vi "grapher.vi"(0 "Eventnum refnum":refnum<vi>, 5 "Frequency refnum":refnum<vi>, 7 "Stop signaller":refnum<class "Signaller.lvclass">, 9 "Polarization refnum":refnum<vi>, 11 "Rate refnum":refnum<vi>) -> ()   [LabVIEW 2015]
uses:
  Motor controller/Signaller/Signaller.lvclass
panel:
  in  "Focus range":dbl=0.1 min=0.001 step=0.1 format="%.3g"
  in  "Focus on current":bool
  in  "Scale for negative":bool
  in  "Scale for positive":bool
  in  "Autoscale polarization":bool=TRUE
  in  "Min polarization":dbl step=0.1 format="%.3g"
  in  "Max polarization":dbl=1.0 step=0.1 format="%.3g"
  in  "Add 1 hour":bool
  in  "1 hour":bool
  in  "30 minutes":bool
  in  "10 minutes":bool
  in  "5 minutes":bool
  in  "1 minute":bool
  in  "Time scale (min)":i64=1 min=1 step=1
  in  "Data output file":path
  out "Data points":i32
  out "Polarization vs frequency":cluster{dbl, dbl}[](graph)
  out "Rate vs time":cluster{"Value":i64, "Value":dbl}[](graph)
  out "Frequency vs time":cluster{"Value":i64, "Value":dbl}[](graph)
  out "Polarization vs time":cluster{i64, dbl}[](graph)
  out "Rate":dbl
  out "Polarization":dbl
  out "Frequency":dbl
  out "Eventnum":i64
  # "Advanced controls"
  # "Graph polarization scale"
  # "Graph time scale"
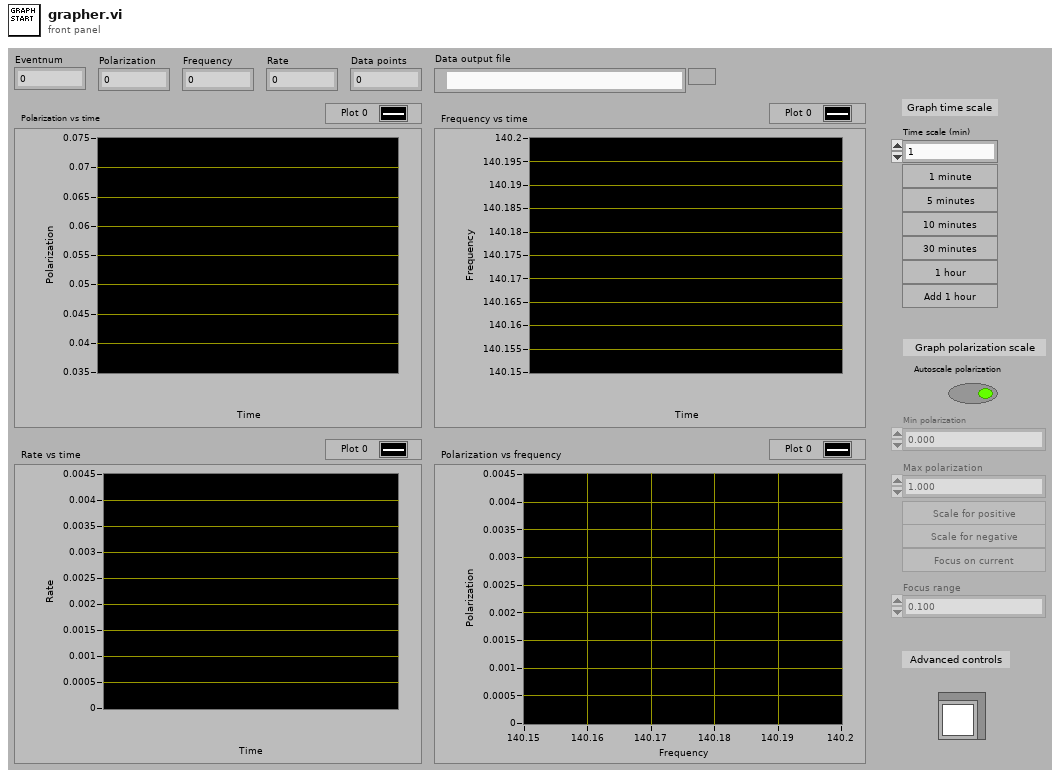
[diagram p1: front panel]
types:
  T1 = typedef "LVRangeTypeDef.ctl" = cluster{"Minimum":dbl, "Maximum":dbl, "Increment":dbl, "Minor Increment":dbl, "Start":dbl}
  T2 = enum8{"Enabled", "Disabled", "Disabled and Grayed Out"}
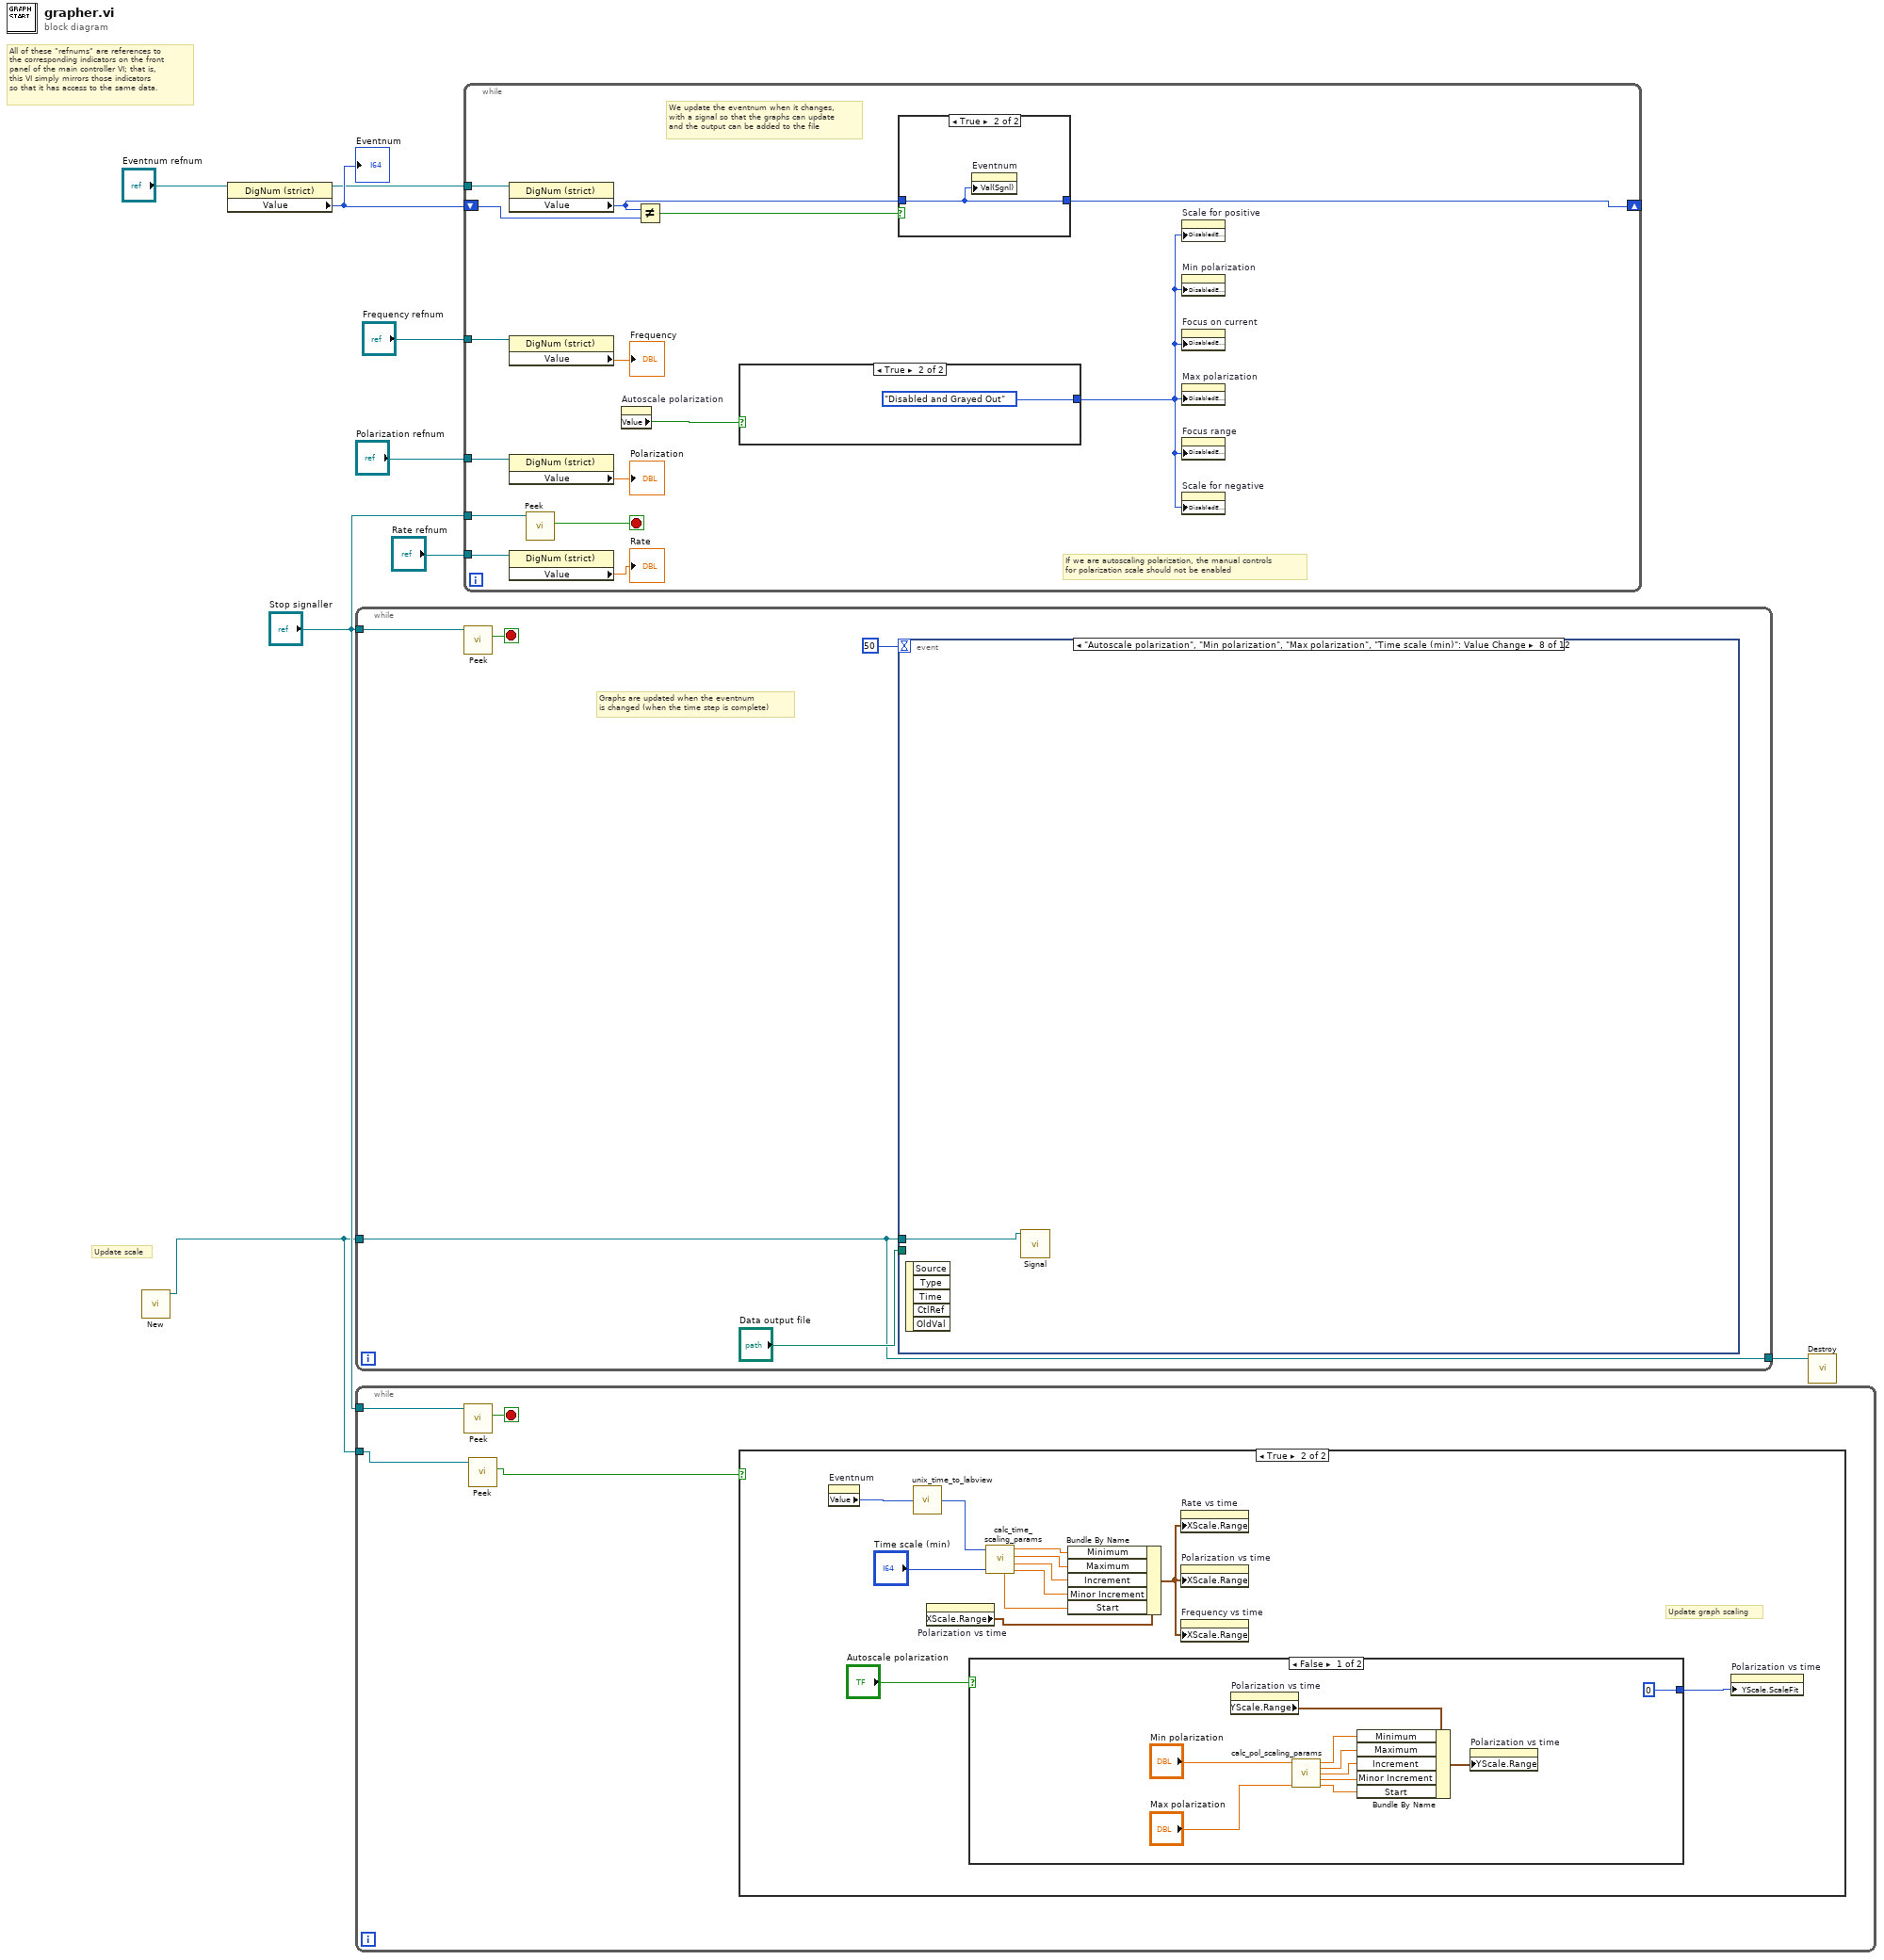
[diagram p0: block diagram]
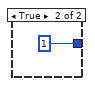
[diagram p3: hidden frame]
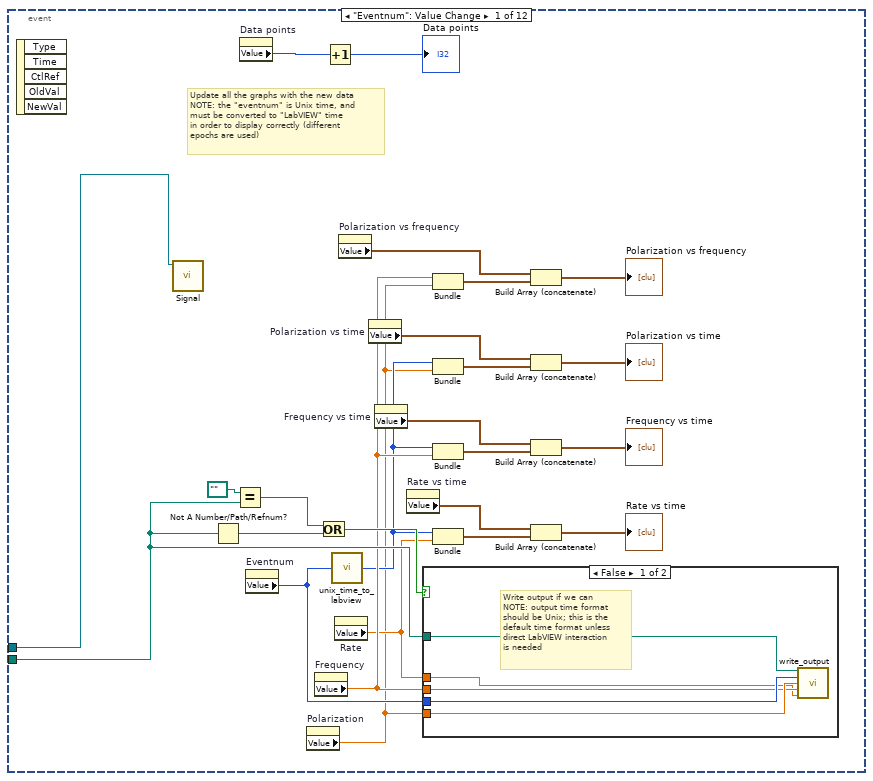
[diagram p4: hidden frame]
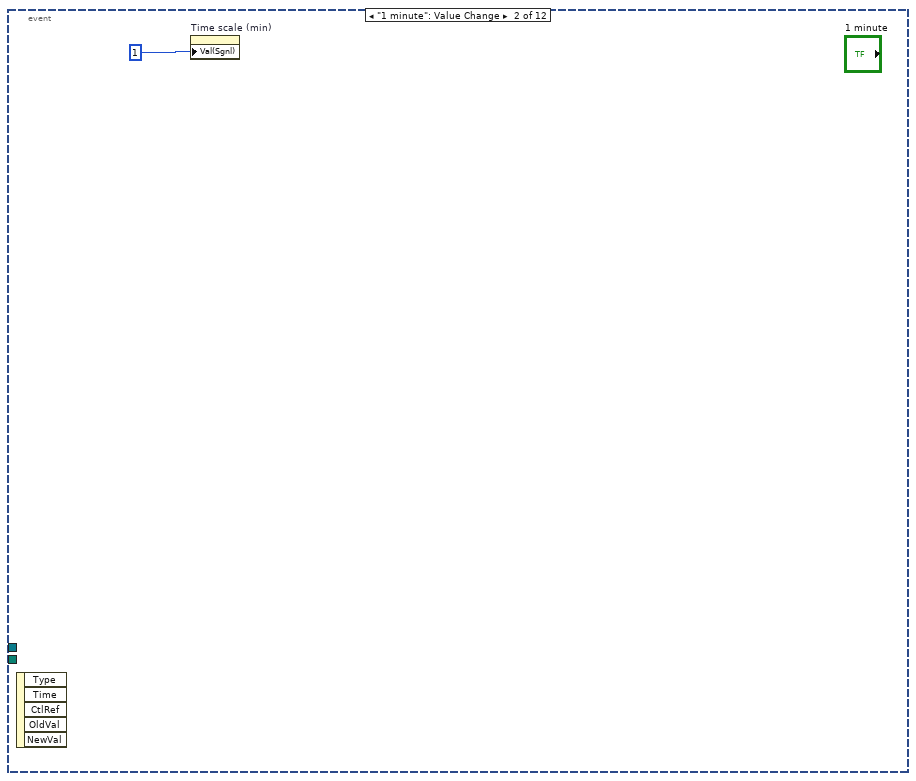
[diagram p6: hidden frame]
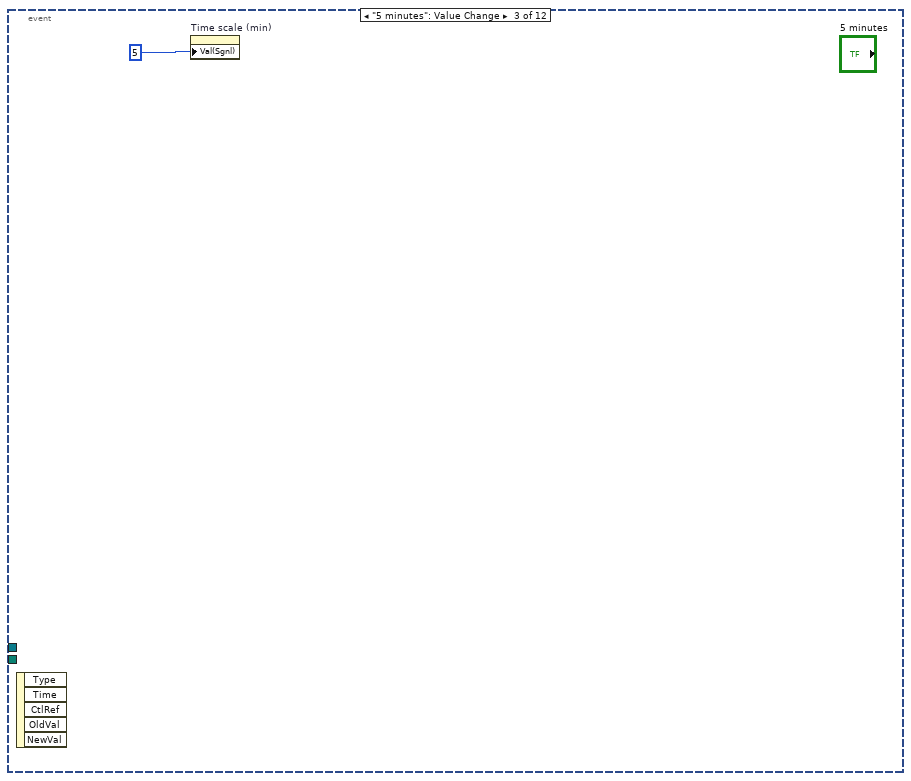
[diagram p7: hidden frame]
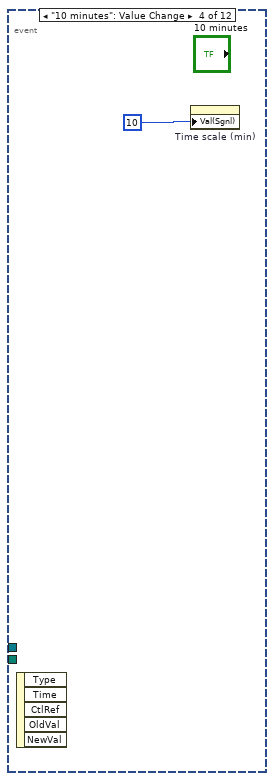
[diagram p8: hidden frame]
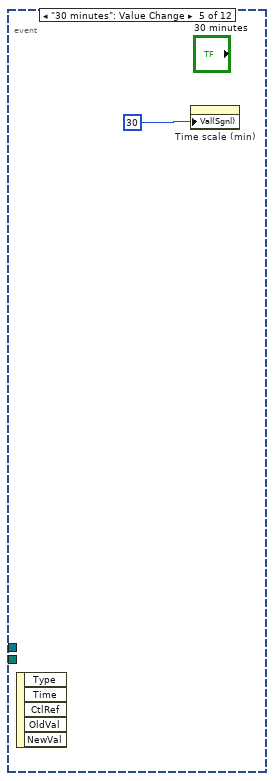
[diagram p9: hidden frame]
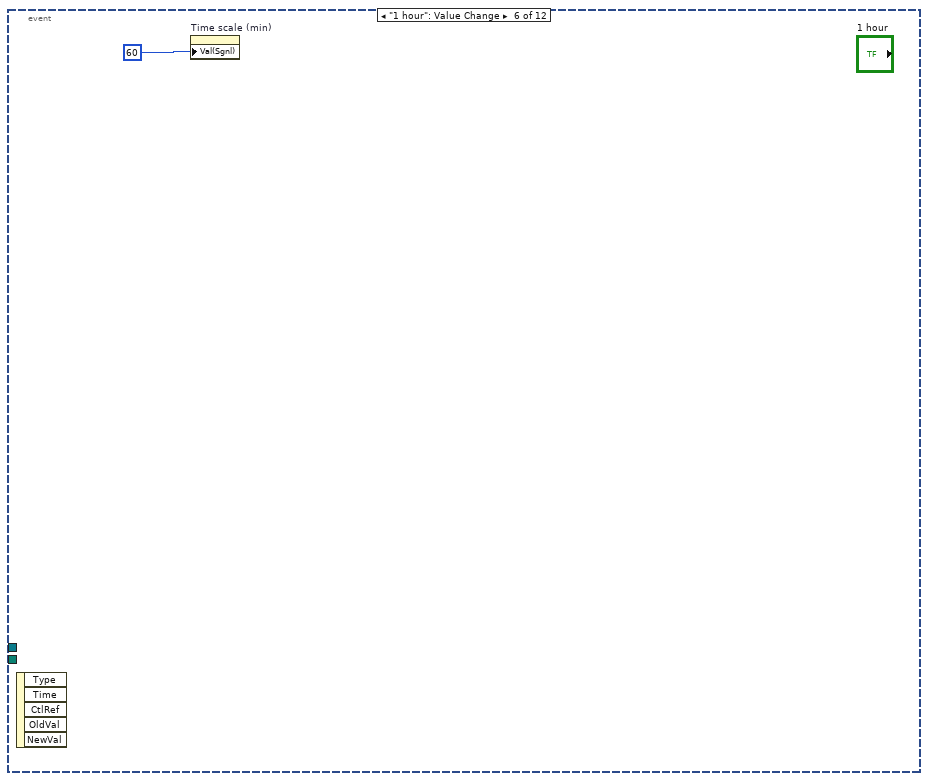
[diagram p10: hidden frame]
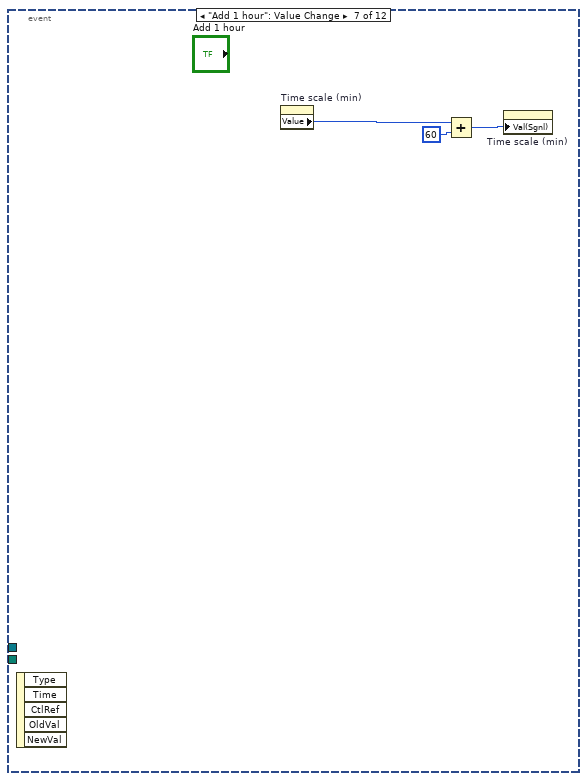
[diagram p11: hidden frame]
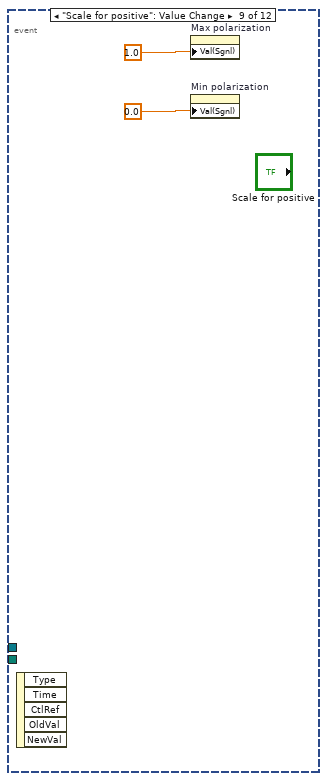
[diagram p12: hidden frame]
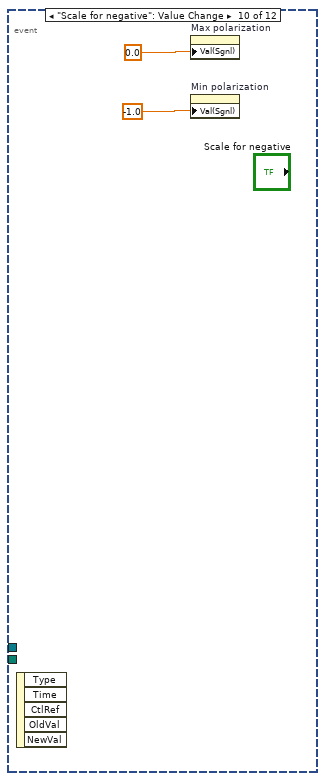
[diagram p13: hidden frame]
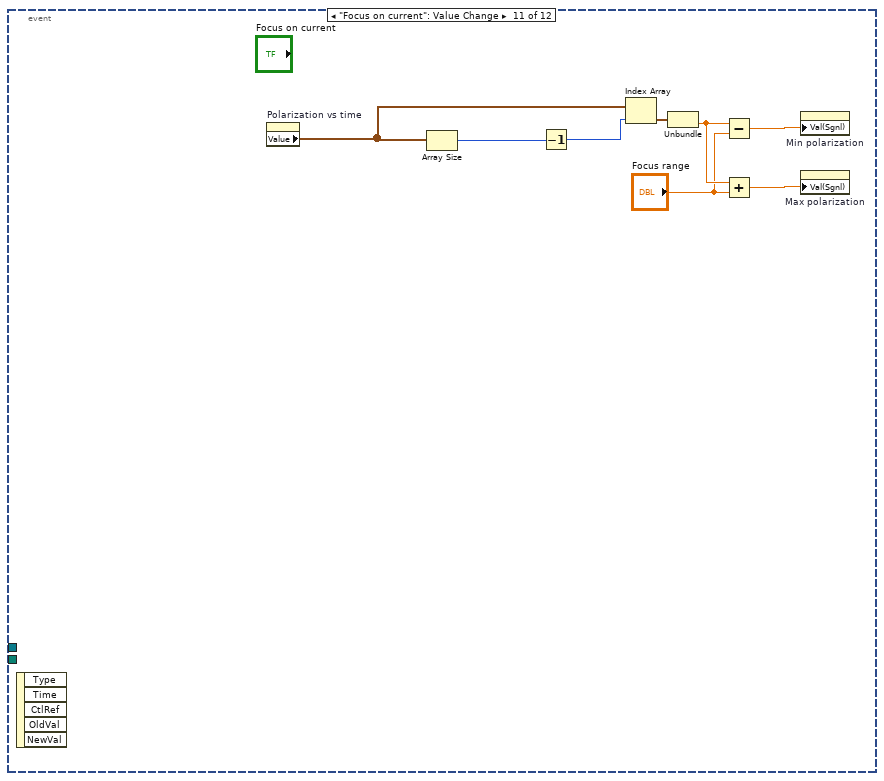
[diagram p14: hidden frame]
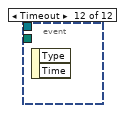
[diagram p15: hidden frame]
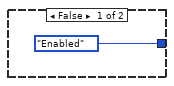
[diagram p16: hidden frame]
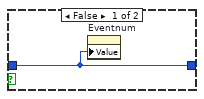
[diagram p17: hidden frame]
diagram:
  # "Update scale"
  # "All of these \"refnums\" are references to\nthe corresponding indicators on the front\npanel of the main controller VI; that is,\nthis VI simply mirrors those indicators\nso that it has access to the same data."
  n1 = call "New.vi"() -> ("Signaller out"=w1:refnum<class "Signaller.lvclass">)  [unwired: 11 in]
  n2 = property class="DigNum (strict)"(reference="Eventnum refnum") -> (reference out=w4:refnum<vi>, "Value"=w5:i64)  [unwired: 1 in, 1 out]
  "Eventnum" <- w5
  n3 = while {
    tunnel: "Stop signaller" -> [w12]
    tunnel: w1 -> [w10]
    tunnel: [w10] -> w3
    stop <- w11 stop-if-true
    # "Graphs are updated when the eventnum\nis changed (when the time step is complete)"
    n4 = call "Peek.vi"("Signaller in"=w12) -> ("Has signal"=w11:bool)  [unwired: 8 in, 2 out]
    n5 = event shown="[7] \"Autoscale polarization\", \"Min polarization\", \"Max polarization\", \"Time scale (min)\": Value Change" {
      selector: _ -> [_ _ _ _ _ _ _ _ _ _ _ _]
      dyn-events: _ -> [_ _ _ _ _ _ _ _ _ _ _ _]
      timeout: 50 -> [_ _ _ _ _ _ _ _ _ _ _ _]
      tunnel: "Data output file" -> [w31 _ _ _ _ _ _ _ _ _ _ _]
      tunnel: w10 -> [w15 _ _ _ _ _ _ w53 _ _ _ _]
      event "Eventnum": Value Change {
        # "Update all the graphs with the new data\nNOTE: the \"eventnum\" is Unix time, and\nmust be converted to \"LabVIEW\" time\nin order to display correctly (different\nepochs are used)"
        n6 = event-data() -> ()  [unwired: 1 in, 5 out]
        n7 = call "Signal.vi"("Signaller in"=w15) -> ()  [unwired: 9 in, 2 out]
        n8 = Not A Number/Path/Refnum?(number/path/refnum=w31) -> (NaN/Path/Refnum?=w35:bool)
        n9 = Equal?(x=path "", y=w31) -> (x = y?=w34:bool)
        n10 = property on="Data points" class="DigNum (strict)"() -> ("Value"=w17:i32)  [unwired: 2 in, 2 out]
        n11 = property on="Eventnum" class="DigNum (strict)"() -> ("Value"=w28:i64)  [unwired: 2 in, 2 out]
        n12 = property on="Polarization" class="DigNum (strict)"() -> ("Value"=w16:dbl)  [unwired: 2 in, 2 out]
        n13 = property on="Frequency" class="DigNum (strict)"() -> ("Value"=w30:dbl)  [unwired: 2 in, 2 out]
        n14 = Or(x=w34, y=w35) -> (x .or. y?=w33:bool)
        n15 = Increment(x=w17) -> (x+1=→"Data points":i32)
        n16 = call "unix_time_to_labview.vi"("Unix time"=w28) -> ("LabVIEW time"=w27:i64)
        n17 = property on="Rate" class="DigNum (strict)"() -> ("Value"=w29:dbl)  [unwired: 2 in, 2 out]
        n18 = property on="Polarization vs frequency" class="XYGraph (strict)"() -> ("Value"=w19:cluster{dbl, dbl}[])  [unwired: 2 in, 2 out]
        n19 = property on="Polarization vs time" class="XYGraph (strict)"() -> ("Value"=w22:cluster{i64, dbl}[])  [unwired: 2 in, 2 out]
        n20 = property on="Frequency vs time" class="XYGraph (strict)"() -> ("Value"=w21:cluster{"Value":i64, "Value":dbl}[])  [unwired: 2 in, 2 out]
        n21 = property on="Rate vs time" class="XYGraph (strict)"() -> ("Value"=w20:cluster{"Value":i64, "Value":dbl}[])  [unwired: 2 in, 2 out]
        n22 = case shown="False" w33 {
          tunnel: w31 -> [w44 _]
          tunnel: w28 -> [w43 _]
          tunnel: w16 -> [w42 _]
          tunnel: w30 -> [w41 _]
          tunnel: w29 -> [w40 _]
          frame False {
            # "Write output if we can\nNOTE: output time format\nshould be Unix; this is the\ndefault time format unless\ndirect LabVIEW interaction\nis needed"
            n23 = call "write_output.vi"("Data output file"=w44, "Time"=w43, "Polarization"=w42, "Frequency"=w41, "Rate"=w40) -> ()  [unwired: 11 in]
          }
          frame True {
          }
        }
        n24 = Bundle("Value"=w30, "Value"=w16) -> (w38:cluster{"Value":dbl, "Value":dbl})  [unwired: 1 in]
        n25 = Bundle("LabVIEW time"=w27, "Value"=w16) -> (w36:cluster{"LabVIEW time":i64, "Value":dbl})  [unwired: 1 in]
        n26 = Bundle("LabVIEW time"=w27, "Value"=w30) -> (w37:cluster{"LabVIEW time":i64, "Value":dbl})  [unwired: 1 in]
        n27 = Bundle("LabVIEW time"=w27, "Value"=w29) -> (w39:cluster{"LabVIEW time":i64, "Value":dbl})  [unwired: 1 in]
        n28 = Build Array (concatenate)(w19, w38) -> (→"Polarization vs frequency":cluster{"Value":dbl, "Value":dbl}[])
        n29 = Build Array (concatenate)(w22, w36) -> (→"Polarization vs time":cluster{"LabVIEW time":i64, "Value":dbl}[])
        n30 = Build Array (concatenate)(w21, w37) -> (→"Frequency vs time":cluster{"LabVIEW time":i64, "Value":dbl}[])
        n31 = Build Array (concatenate)(w20, w39) -> (→"Rate vs time":cluster{"LabVIEW time":i64, "Value":dbl}[])
      }
      event "1 minute": Value Change {
        n32 = event-data() -> ()  [unwired: 1 in, 5 out]
        n33 = property on="Time scale (min)" class="DigNum (strict)"("Val(Sgnl)"=i64 1 ("Value (Signaling)")) -> ()  [unwired: 2 in, 2 out]
      }
      event "5 minutes": Value Change {
        n34 = event-data() -> ()  [unwired: 1 in, 5 out]
        n35 = property on="Time scale (min)" class="DigNum (strict)"("Val(Sgnl)"=i64 5 ("Value (Signaling)")) -> ()  [unwired: 2 in, 2 out]
      }
      event "10 minutes": Value Change {
        n36 = event-data() -> ()  [unwired: 1 in, 5 out]
        n37 = property on="Time scale (min)" class="DigNum (strict)"("Val(Sgnl)"=i64 10 ("Value (Signaling)")) -> ()  [unwired: 2 in, 2 out]
      }
      event "30 minutes": Value Change {
        n38 = event-data() -> ()  [unwired: 1 in, 5 out]
        n39 = property on="Time scale (min)" class="DigNum (strict)"("Val(Sgnl)"=i64 30 ("Value (Signaling)")) -> ()  [unwired: 2 in, 2 out]
      }
      event "1 hour": Value Change {
        n40 = event-data() -> ()  [unwired: 1 in, 5 out]
        n41 = property on="Time scale (min)" class="DigNum (strict)"("Val(Sgnl)"=i64 60 ("Value (Signaling)")) -> ()  [unwired: 2 in, 2 out]
      }
      event "Add 1 hour": Value Change {
        n42 = event-data() -> ()  [unwired: 1 in, 5 out]
        n43 = property on="Time scale (min)" class="DigNum (strict)"() -> ("Value"=w52:i64)  [unwired: 2 in, 2 out]
        n44 = Add(x=w52, y=i64 60) -> (x+y=w50:i64)
        n45 = property on="Time scale (min)" class="DigNum (strict)"("Val(Sgnl)"=w50) -> ()  [unwired: 2 in, 2 out]
      }
      event "Autoscale polarization", "Min polarization", "Max polarization", "Time scale (min)": Value Change {
        n46 = event-data() -> ()  [unwired: 1 in, 5 out]
        n47 = call "Signal.vi"("Signaller in"=w53) -> ()  [unwired: 9 in, 2 out]
      }
      event "Scale for positive": Value Change {
        n48 = event-data() -> ()  [unwired: 1 in, 5 out]
        n49 = property on="Max polarization" class="DigNum (strict)"("Val(Sgnl)"=1.0 ("Value (Signaling)")) -> ()  [unwired: 2 in, 2 out]
        n50 = property on="Min polarization" class="DigNum (strict)"("Val(Sgnl)"=0.0 ("Value (Signaling)")) -> ()  [unwired: 2 in, 2 out]
      }
      event "Scale for negative": Value Change {
        n51 = event-data() -> ()  [unwired: 1 in, 5 out]
        n52 = property on="Max polarization" class="DigNum (strict)"("Val(Sgnl)"=0.0 ("Value (Signaling)")) -> ()  [unwired: 2 in, 2 out]
        n53 = property on="Min polarization" class="DigNum (strict)"("Val(Sgnl)"=-1.0 ("Value (Signaling)")) -> ()  [unwired: 2 in, 2 out]
      }
      event "Focus on current": Value Change {
        n54 = event-data() -> ()  [unwired: 1 in, 5 out]
        n55 = property on="Polarization vs time" class="XYGraph (strict)"() -> ("Value"=w65:cluster{i64, dbl}[])  [unwired: 2 in, 2 out]
        n56 = Array Size(array=w65) -> (size(s)=w64:i32)
        n57 = Decrement(x=w64) -> (x-1=w63:i32)
        n58 = Index Array(array=w65, index=w63) -> (element=w62:cluster{i64, dbl})
        n59 = Unbundle(w62) -> (w59:dbl)  [unwired: 1 out]
        n60 = Subtract(x=w59, y="Focus range") -> (x-y=w60:dbl)
        n61 = Add(x=w59, y="Focus range") -> (x+y=w61:dbl)
        n62 = property on="Min polarization" class="DigNum (strict)"("Val(Sgnl)"=w60) -> ()  [unwired: 2 in, 2 out]
        n63 = property on="Max polarization" class="DigNum (strict)"("Val(Sgnl)"=w61) -> ()  [unwired: 2 in, 2 out]
      }
      event Timeout {
        n64 = event-data() -> ()  [unwired: 1 in, 2 out]
      }
    }
  }
  n65 = while {
    tunnel: w1 -> [w67]
    tunnel: "Stop signaller" -> [w69]
    stop <- w68 stop-if-true
    n66 = call "Peek.vi"("Signaller in"=w69) -> ("Has signal"=w68:bool)  [unwired: 8 in, 2 out]
    n67 = call "Peek.vi"("Signaller in"=w67) -> ("Has signal"=w66:bool)  [unwired: 8 in, 2 out]
    n68 = case shown="True" w66 {
      frame False {
      }
      frame True {
        # "Update graph scaling"
        n69 = property on="Eventnum" class="DigNum (strict)"() -> ("Value"=w73:i64)  [unwired: 2 in, 2 out]
        n70 = call "unix_time_to_labview.vi"("Unix time"=w73) -> ("LabVIEW time"=w72:i64)
        n71 = property on="Polarization vs time" class="XYGraph (strict)"() -> ("XScale.Range"=w81:T1)  [unwired: 2 in, 2 out]
        n72 = case shown="False" "Autoscale polarization" {
          tunnel: [u8 0 ("Y Scale.Scale Fit") u8 1 ("Y Scale.Scale Fit")] -> w70
          frame False {
            n73 = property on="Polarization vs time" class="XYGraph (strict)"() -> ("YScale.Range"=w89:T1)  [unwired: 2 in, 2 out]
            n74 = call "calc_pol_scaling_params.vi"("Min polarization"="Min polarization", "Max polarization"="Max polarization") -> ("Minimum"=w87:dbl, "Maximum"=w86:dbl, "Increment"=w85:dbl, "Minor increment"=w84:dbl, "Start"=w83:dbl)  [unwired: 9 in]
            n75 = Bundle By Name(cluster=w89, "Minimum"=w87, "Maximum"=w86, "Increment"=w85, "Minor Increment"=w84, "Start"=w83) -> (w88:T1)
            n76 = property on="Polarization vs time" class="XYGraph (strict)"("YScale.Range"=w88) -> ()  [unwired: 2 in, 2 out]
          }
          frame True {
          }
        }
        n77 = call "calc_time_scaling_params.vi"("Time"=w72, "Time scale (minutes)"="Time scale (min)") -> ("Minimum"=w78:dbl, "Maximum"=w77:dbl, "Increment"=w76:dbl, "Minor increment"=w75:dbl, "Start"=w80:dbl)  [unwired: 1 in]
        n78 = Bundle By Name(cluster=w81, "Minimum"=w78, "Maximum"=w77, "Increment"=w76, "Minor Increment"=w75, "Start"=w80) -> (w79:T1)
        n79 = property on="Rate vs time" class="XYGraph (strict)"("XScale.Range"=w79) -> ()  [unwired: 2 in, 2 out]
        n80 = property on="Polarization vs time" class="XYGraph (strict)"("XScale.Range"=w79) -> ()  [unwired: 2 in, 2 out]
        n81 = property on="Frequency vs time" class="XYGraph (strict)"("XScale.Range"=w79) -> ()  [unwired: 2 in, 2 out]
        n82 = property on="Polarization vs time" class="XYGraph (strict)"("YScale.ScaleFit"=w70) -> ()  [unwired: 2 in, 2 out]
      }
    }
  }
  n83 = while {
    tunnel: "Polarization refnum" -> [w107]
    tunnel: "Frequency refnum" -> [w106]
    tunnel: w4 -> [w105]
    tunnel: "Rate refnum" -> [w104]
    shift-right: [w100] -> _
    shift-left: w5 -> [w101]
    tunnel: "Stop signaller" -> [w96]
    stop <- w95 stop-if-true
    # "We update the eventnum when it changes,\nwith a signal so that the graphs can update\nand the output can be added to the file"
    # "If we are autoscaling polarization, the manual controls\nfor polarization scale should not be enabled"
    n84 = property class="DigNum (strict)"(reference=w105) -> ("Value"=w102:i64)  [unwired: 1 in, 2 out]
    n85 = property class="DigNum (strict)"(reference=w106) -> ("Value"=→"Frequency":dbl)  [unwired: 1 in, 2 out]
    n86 = property class="DigNum (strict)"(reference=w107) -> ("Value"=→"Polarization":dbl)  [unwired: 1 in, 2 out]
    n87 = property class="DigNum (strict)"(reference=w104) -> ("Value"=→"Rate":dbl)  [unwired: 1 in, 2 out]
    n88 = call "Peek.vi"("Signaller in"=w96) -> ("Has signal"=w95:bool)  [unwired: 8 in, 2 out]
    n89 = property on="Autoscale polarization" class="Bool (strict)"() -> ("Value"=w94:bool)  [unwired: 2 in, 2 out]
    n90 = Not Equal?(x=w102, y=w101) -> (x != y?=w103:bool)
    n91 = case shown="True" w94 {
      tunnel: [T2."Enabled" ("Disabled") T2."Disabled and Grayed Out" ("Disabled")] -> w93
      frame False {
      }
      frame True {
      }
    }
    n92 = case shown="True" w103 {
      tunnel: w102 -> [w110 w111]
      tunnel: [w110 w111] -> w100
      frame False {
        n93 = property on="Eventnum" class="DigNum (strict)"("Value"=w110) -> ()  [unwired: 2 in, 2 out]
      }
      frame True {
        n94 = property on="Eventnum" class="DigNum (strict)"("Val(Sgnl)"=w111) -> ()  [unwired: 2 in, 2 out]
      }
    }
    n95 = property on="Scale for positive" class="Bool"("DisabledEnum"=w93) -> ()  [unwired: 2 in, 2 out]
    n96 = property on="Min polarization" class="DigNum (strict)"("DisabledEnum"=w93) -> ()  [unwired: 2 in, 2 out]
    n97 = property on="Focus on current" class="Bool"("DisabledEnum"=w93) -> ()  [unwired: 2 in, 2 out]
    n98 = property on="Max polarization" class="DigNum (strict)"("DisabledEnum"=w93) -> ()  [unwired: 2 in, 2 out]
    n99 = property on="Focus range" class="DigNum (strict)"("DisabledEnum"=w93) -> ()  [unwired: 2 in, 2 out]
    n100 = property on="Scale for negative" class="Bool"("DisabledEnum"=w93) -> ()  [unwired: 2 in, 2 out]
  }
  n101 = call "Destroy.vi"("Signaller in"=w3) -> ()  [unwired: 10 in, 1 out]
